vi "Serial_RS232.vi"() -> ()   [LabVIEW 2020]
uses:
  <vilib>/Instr/_visa.llb/VISA Configure Serial Port (Instr).vi
panel:
  in  "end Program":bool
  out "error out 2":errorcluster
  in  "Cluster":T1
  in  "control":bool
  out "*(type *) &x":T2
  in  "baud rate (115200)":u32=9600
  in  "VISA PortName":refnum<visa-resource-name>
  out "error out":errorcluster
  out "read buffer":string
  in  "write buffer":string
  in  "stop":bool
  in  "baud rate (9600)":u32=9600
  in  "VISA resource name":refnum<visa-resource-name>
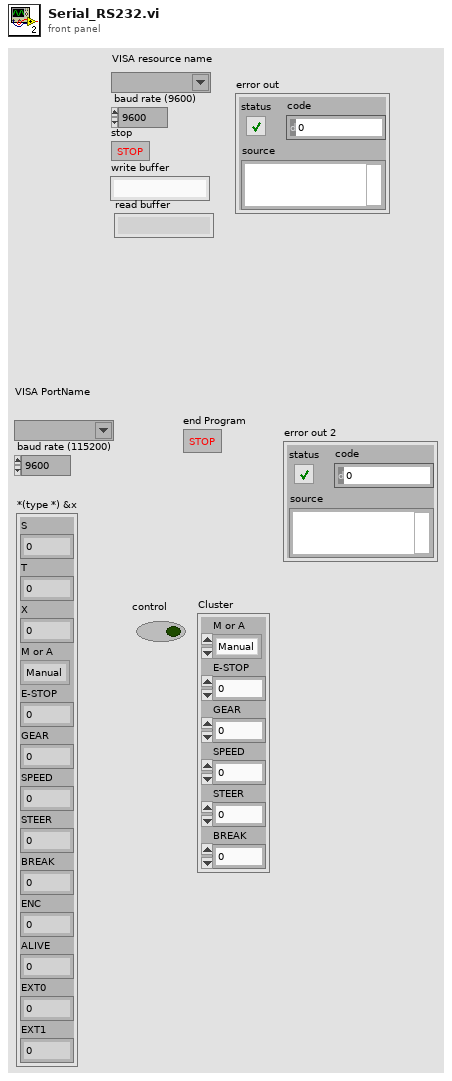
[diagram p1: front panel]
types:
  T1 = cluster{"M or A":enum16{"Manual", "Auto"}, "E-STOP":u8, "GEAR":u8, "SPEED":u16, "STEER":i16, "BREAK":u8}
  T2 = cluster{"S":u8, "T":u8, "X":u8, "M or A":enum16{"Manual", "Auto"}, "E-STOP":u8, "GEAR":u8, "SPEED":u16, "STEER":i16, "BREAK":u8, "ENC":i32, "ALIVE":u8, "EXT0":u8, "EXT1":u8}
  T3 = cluster{"S":u8, "T":u8, "X":u8, "M or A":enum16{"Manual", "Auto"}, "E-STOP":u8, "GEAR":u8, "SPEED":u16, "STEER":i16, "BREAK":u8, "ALIVE":u8, "EXT0":u8, "EXT1":u8}
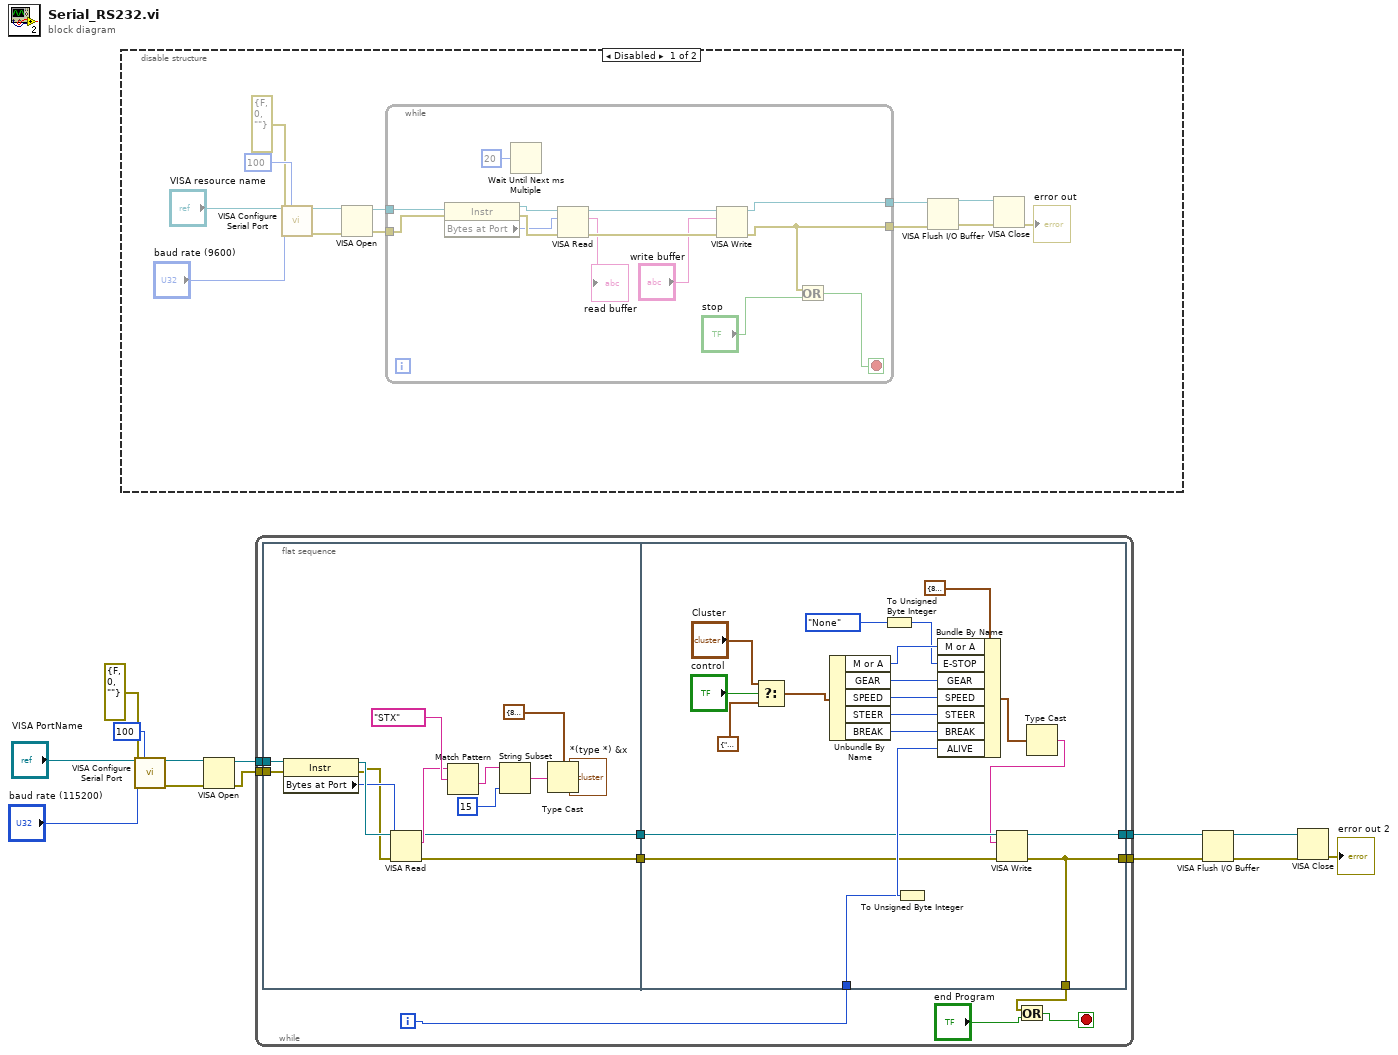
[diagram p0: block diagram]
diagram:
  n1 = disable-structure shown="Disabled" {
    frame Disabled {
      n2 = call-poly "VISA Configure Serial Port"("VISA resource name"="VISA resource name", "timeout (10sec)"=u32 100, "baud rate (9600)"="baud rate (9600)", "error in (no error)"=errorcluster {"status"=FALSE, "code"=0, "source"=""}) -> ("VISA resource name out"=w23:refnum<visa-resource-name>, "error out"=w22:errorcluster)  [unwired: 10 in]
      n3 = VISA Open(error in (no error)=w22, VISA resource name=w23) -> (VISA resource name=w20:refnum<visa-resource-name>, error out=w19:errorcluster)  [unwired: 3 in]
      n4 = while {
        tunnel: w20 -> [w40]
        tunnel: w19 -> [w39]
        tunnel: [w32] -> w16
        tunnel: [w30] -> w15
        stop <- w29 stop-if-true
        n5 = property class="Instr"(reference=w40, error in=w39) -> (reference out=w38:refnum<visa-resource-name>, error out=w37:errorcluster, "Bytes at Port"=w36:u32)
        n6 = Wait Until Next ms Multiple(millisecond multiple=u32 20) -> ()  [unwired: 1 out]
        n7 = VISA Read(VISA resource name=w38, byte count=w36, error in (no error)=w37) -> (VISA resource name out=w35:refnum<visa-resource-name>, read buffer=→"read buffer":string, error out=w34:errorcluster)  [unwired: 1 out]
        n8 = VISA Write(VISA resource name=w35, write buffer="write buffer", error in (no error)=w34) -> (VISA resource name out=w32:refnum<visa-resource-name>, error out=w30:errorcluster)  [unwired: 1 out]
        n9 = Or(x=w30, y="stop") -> (x .or. y?=w29:bool)
      }
      n10 = VISA Flush I/O Buffer(VISA resource name=w16, error in (no error)=w15) -> (VISA resource name out=w18:refnum<visa-resource-name>, error out=w17:errorcluster)  [unwired: 1 in]
      n11 = VISA Close(VISA resource name=w18, error in (no error)=w17) -> (error out=→"error out":errorcluster)
    }
    frame Enabled {
    }
  }
  n12 = call-poly "VISA Configure Serial Port"("VISA resource name"="VISA PortName", "timeout (10sec)"=u32 100, "baud rate (9600)"="baud rate (115200)", "error in (no error)"=errorcluster {"status"=FALSE, "code"=0, "source"=""}) -> ("VISA resource name out"=w9:refnum<visa-resource-name>, "error out"=w10:errorcluster)  [unwired: 10 in]
  n13 = VISA Open(error in (no error)=w10, VISA resource name=w9) -> (VISA resource name=w7:refnum<visa-resource-name>, error out=w6:errorcluster)  [unwired: 3 in]
  n14 = while {
    tunnel: w7 -> [w50]
    tunnel: w6 -> [w49]
    tunnel: [w45] -> w2
    tunnel: [w44] -> w1
    i -> [w48]
    stop <- w42 stop-if-true
    n15 = flat-sequence {
      tunnel: w50 -> [w64]
      tunnel: w49 -> [w63]
      tunnel: [w52] -> w47
      tunnel: [w51] -> w46
      tunnel: w48 -> [w82]
      tunnel: w47 -> [w70]
      tunnel: w46 -> [w69]
      tunnel: [w68] -> w45
      tunnel: [w65] -> w44
      tunnel: [w65] -> w41
      frame #0 {
        n16 = property class="Instr"(reference=w64, error in=w63) -> (reference out=w56:refnum<visa-resource-name>, error out=w54:errorcluster, "Bytes at Port"=w55:u32)
        n17 = VISA Read(VISA resource name=w56, byte count=w55, error in (no error)=w54) -> (VISA resource name out=w52:refnum<visa-resource-name>, read buffer=w53:string, error out=w51:errorcluster)  [unwired: 1 out]
        n18 = Match Pattern(string=w53, regular expression="STX") -> (after substring=w61:string)  [unwired: 1 in, 3 out]
        n19 = String Subset(string=w61, length (rest)=15 ("length (rest)")) -> (substring=w59:string)  [unwired: 1 in]
        n20 = Type Cast(type=T2 {"S"=83, "T"=84, "X"=88, "M or A"=enum."Manual", "E-STOP"=0, "GEAR"=0, "SPEED"=0, "STEER"=0, "BREAK"=0, "ENC"=0, "ALIVE"=0, "EXT0"=0, "EXT1"=0}, x=w59) -> (*(type *) &x=→"*(type *) &x":T2)
      }
      frame #1 {
        n21 = Select(t="Cluster", s="control", f=T1 {"M or A"=enum."Manual", "E-STOP"=0, "GEAR"=1, "SPEED"=0, "STEER"=0, "BREAK"=150}) -> (s? t:f=w76:T1)
        n22 = Unbundle By Name(w76) -> ("M or A"=w81:enum16{"Manual", "Auto"}, "GEAR"=w80:u8, "SPEED"=w79:u16, "STEER"=w78:i16, "BREAK"=w77:u8)
        n23 = To Unsigned Byte Integer(number=enum8{"None", "Emergency-STOP"}."None") -> (unsigned 8bit integer=w71:u8)
        n24 = To Unsigned Byte Integer(number=w82) -> (unsigned 8bit integer=w83:u8)
        n25 = Bundle By Name(cluster=T3 {"S"=83, "T"=84, "X"=88, "M or A"=enum."Manual", "E-STOP"=0, "GEAR"=0, "SPEED"=0, "STEER"=0, "BREAK"=0, "ALIVE"=0, "EXT0"=0, "EXT1"=0}, "M or A"=w81, "E-STOP"=w71, "GEAR"=w80, "SPEED"=w79, "STEER"=w78, "BREAK"=w77, "ALIVE"=w83) -> (w67:T3)
        n26 = Type Cast(x=w67) -> (*(type *) &x=w66:string)  [unwired: 1 in]
        n27 = VISA Write(VISA resource name=w70, write buffer=w66, error in (no error)=w69) -> (VISA resource name out=w68:refnum<visa-resource-name>, error out=w65:errorcluster)  [unwired: 1 out]
      }
    }
    n28 = Or(x=w41, y="end Program") -> (x .or. y?=w42:bool)
  }
  n29 = VISA Flush I/O Buffer(VISA resource name=w2, error in (no error)=w1) -> (VISA resource name out=w5:refnum<visa-resource-name>, error out=w4:errorcluster)  [unwired: 1 in]
  n30 = VISA Close(VISA resource name=w5, error in (no error)=w4) -> (error out=→"error out 2":errorcluster)
